vi "Edit Control File.vi"(0 "Control File":path=path "D:/Workspace/measurementlink-labview/Source/SolutionBuilder/Proto/builds/Build/BuildPlugin/control/control", 5 "MeasName":string, 9 "Version":string, 11 "error in (no error)":errorcluster) -> (15 "error out":errorcluster)   [LabVIEW 2021, in "Measurement Builder.lvlib"]
uses:
  Measurement Builder.lvlib
  controls/Config File Operations.ctl
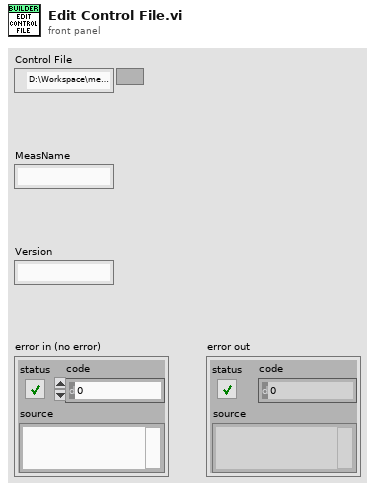
[diagram p1: front panel]
types:
  T1 = typedef "Measurement Builder.lvlib/Config File Operations.ctl" = enum16{"Read", "Write"}
  T2 = enum16{"open", "replace", "create", "open or create", "replace or create", "replace or create with confirmation"}
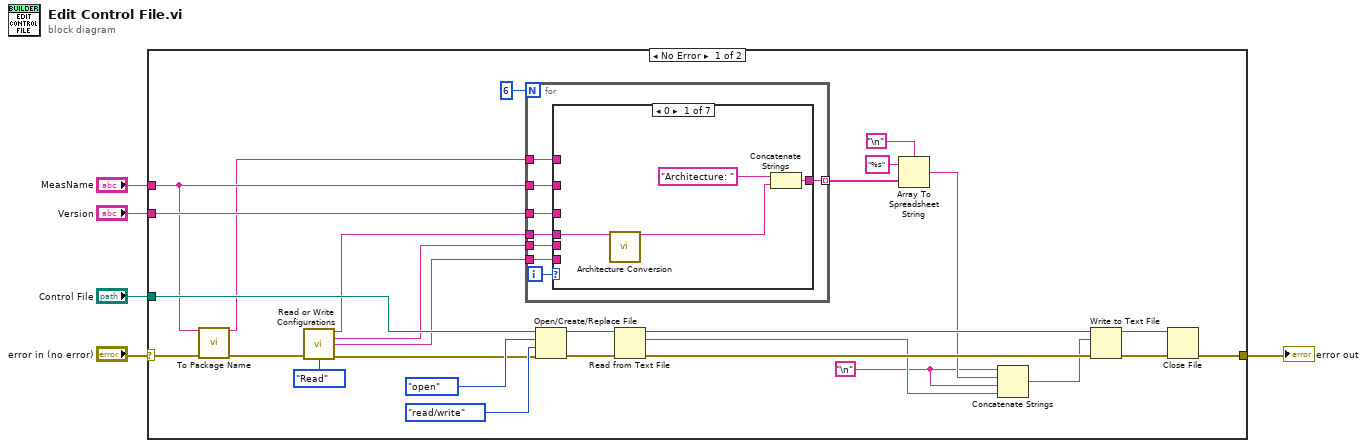
[diagram p0: block diagram]
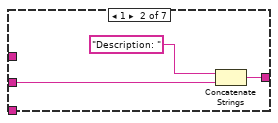
[diagram p2: hidden frame]
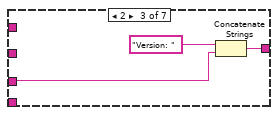
[diagram p3: hidden frame]
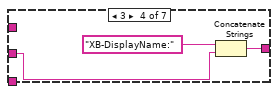
[diagram p4: hidden frame]
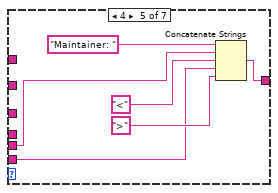
[diagram p5: hidden frame]
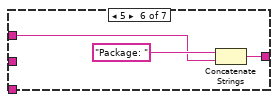
[diagram p6: hidden frame]
diagram:
  n1 = case shown="No Error" "error in (no error)" {
    selector: "error in (no error)" -> [w8 w64]
    tunnel: "Control File" -> [w33 _]
    tunnel: [w30 w64] -> w3
    tunnel: "MeasName" -> [w7 _]
    tunnel: "Version" -> [w10 _]
    frame No Error {
      w16 = "\n"
      n2 = call "To Package Name.vi"("Package Name"=w7, "error in (no error)"=w8) -> ("Valid Package Name"=w6:string, "error out"=w9:errorcluster)  [unwired: 12 in]
      n3 = call "Read or Write Configurations.vi"("error in (no error)"=w9, "Operation"=Config_File_Operations."Read") -> ("Architecture OUT"=w13:string, "Maintainer OUT"=w12:string, "Email OUT"=w11:string, "error out"=w15:errorcluster)  [unwired: 10 in]
      n4 = for {
        N: 6 -> [_]
        tunnel: [w40] -> w28 mode=indexing
        tunnel: w13 -> [w39]
        tunnel: w7 -> [w38]
        tunnel: w10 -> [w37]
        tunnel: w12 -> [w36]
        tunnel: w11 -> [w35]
        tunnel: w6 -> [w34]
        i -> [w41]
        n5 = case shown="0" w41 {
          tunnel: [w44 w47 w50 w53 w59 w62 _] -> w40
          tunnel: w39 -> [w43 _ _ _ _ _ _]
          tunnel: w38 -> [_ w46 _ w52 _ _ _]
          tunnel: w37 -> [_ _ w49 _ _ _ _]
          tunnel: w36 -> [_ _ _ _ w56 _ _]
          tunnel: w35 -> [_ _ _ _ w55 _ _]
          tunnel: w34 -> [_ _ _ _ _ w61 _]
          frame 0 {
            n6 = call "Architecture Conversion.vi"("Arch In"=w43) -> ("Arch OUT"=w42:string)  [unwired: 14 in]
            n7 = Concatenate Strings("Architecture: " ("regular expression"), w42) -> (w44:string)
          }
          frame 1 {
            n8 = Concatenate Strings("Description: " ("regular expression"), w46) -> (w47:string)
          }
          frame 2 {
            n9 = Concatenate Strings("Version: " ("regular expression"), w49) -> (w50:string)
          }
          frame 3 {
            n10 = Concatenate Strings("XB-DisplayName:" ("regular expression"), w52) -> (w53:string)
          }
          frame 4 {
            n11 = Concatenate Strings("Maintainer: " ("regular expression"), w56, "<" ("string"), w55, ">" ("string")) -> (w59:string)
          }
          frame 5 {
            n12 = Concatenate Strings("Package: " ("regular expression"), w61) -> (w62:string)
          }
          frame Default {
          }
        }
      }
      n13 = Open/Create/Replace File(file path (use dialog)=w33, error in=w15, operation (0:open)=T2."open", access (0:read/write)=enum16{"read/write", "read-only", "write-only"}."read/write") -> (refnum out=w23:refnum<file>, error out=w21:errorcluster)  [unwired: 2 in, 1 out]
      n14 = Read from Text File(file (use dialog)=w23, error in=w21) -> (refnum out=w22:refnum<file>, text=w17:string, error out=w20:errorcluster)  [unwired: 2 in, 1 out]
      n15 = Array To Spreadsheet String(delimiter (Tab)="\n", array=w28, 3:"%s" ("format string")) -> (spreadsheet string=w19:string)
      n16 = Concatenate Strings(w16, w19, w16, w17) -> (w18:string)
      n17 = Write to Text File(file (use dialog)=w22, text=w18, error in=w20) -> (refnum out=w24:refnum<file>, error out=w25:errorcluster)  [unwired: 1 in, 1 out]
      n18 = Close File(refnum=w24, error in=w25) -> (error out=w30:errorcluster)  [unwired: 1 out]
    }
    frame Error {
    }
  }
  "error out" <- w3
